vi "Max Nr of Scalar Channels Test.vi"() -> ()   [LabVIEW 2018]
panel:
  in  "I16 4":i16
  in  "I8 4":i8
  in  "I64 4":i64
  in  "I32 4":i32
  out "I16 out 4":i16
  out "I8 out 4":i8
  out "I32 out 4":i32
  in  "Group1.I16 3":i16
  in  "Group1.I8 3":i8
  in  "Group1.I64 3":i64
  in  "Group1.I32 3":i32
  in  "Group1.U16 3":u16
  in  "Group1.U8 3":u8
  in  "Group1.U64 3":u64
  in  "Group1.U32 3":u32
  in  "Group1.SGL 3":sgl
  in  "Group2.Boolean 3":bool
  out "Group1.I16 out 3":i16
  out "Group1.I8 out 3":i8
  out "Group1.I64 out 3":i64
  out "Group1.I32 out 3":i32
  out "Group1.U16 out 3":u16
  out "Group1.U8 out 3":u8
  out "Group1.U64 out 3":u64
  out "Group1.U32 out 3":u32
  out "Group1.SGL out 3":sgl
  out "Group2.Boolean out 3":bool
  in  "Group2.FXP24.5 3":fxp<+/-,24,5>
  in  "Group2.FXP16.5 3":fxp<+/-,16,5>
  in  "Group2.FXP32.8 3":fxp<+/-,32,8>
  in  "Group2.FXP64.32 3":fxp<+/-,64,32>
  out "Group2.FXP24.5 out 3":fxp<+/-,24,5>
  out "Group2.FXP16.5 out 3":fxp<+/-,16,5>
  out "Group2.FXP32.8 out 3":fxp<+/-,32,8>
  out "Group2.FXP64.32 out 3":fxp<+/-,64,32>
  in  "Group2.FXP16.7 3":fxp<+/-,16,7>
  out "Group2.FXP16.7 out 3":fxp<+/-,16,7>
  in  "Group2.FXP20.5 3":fxp<+/-,20,5>
  out "Group2.FXP20.5 out 3":fxp<+/-,20,5>
  in  "Group2.FXP27.5 3":fxp<+/-,27,5>
  out "Group2.FXP27.5 out 3":fxp<+/-,27,5>
  in  "Group2.FXP32.16 3":fxp<+/-,32,16>
  out "Group2.FXP32.16 out 3":fxp<+/-,32,16>
  in  "Group2.FXP16.3 3":fxp<+,16,3>
  out "Group2.FXP16.3 out 3":fxp<+,16,3>
  in  "Group2.FXP18.3 3":fxp<+,18,3>
  out "Group2.FXP18.3 out 3":fxp<+,18,3>
  in  "I16 3":i16
  in  "I8 3":i8
  in  "I64 3":i64
  in  "I32 3":i32
  in  "U16 3":u16
  in  "U8 3":u8
  in  "U64 3":u64
  in  "U32 3":u32
  in  "SGL 3":sgl
  in  "Boolean 3":bool
  out "I16 out 3":i16
  out "I8 out 3":i8
  out "I64 out 3":i64
  out "I32 out 3":i32
  out "U16 out 3":u16
  out "U8 out 3":u8
  out "U64 out 3":u64
  out "U32 out 3":u32
  out "SGL out 3":sgl
  out "Boolean out 3":bool
  in  "FXP24.5 3":fxp<+/-,24,5>
  in  "FXP16.5 3":fxp<+/-,16,5>
  in  "FXP32.8 3":fxp<+/-,32,8>
  in  "FXP64.32 3":fxp<+/-,64,32>
  out "FXP24.5 out 3":fxp<+/-,24,5>
  out "FXP16.5 out 3":fxp<+/-,16,5>
  out "FXP32.8 out 3":fxp<+/-,32,8>
  out "FXP64.32 out 3":fxp<+/-,64,32>
  in  "FXP16.7 3":fxp<+/-,16,7>
  out "FXP16.7 out 3":fxp<+/-,16,7>
  in  "FXP20.5 3":fxp<+/-,20,5>
  out "FXP20.5 out 3":fxp<+/-,20,5>
  in  "FXP27.5 3":fxp<+/-,27,5>
  out "FXP27.5 out 3":fxp<+/-,27,5>
  in  "FXP32.16 3":fxp<+/-,32,16>
  out "FXP32.16 out 3":fxp<+/-,32,16>
  in  "FXP16.3 3":fxp<+,16,3>
  out "FXP16.3 out 3":fxp<+,16,3>
  in  "FXP18.3 3":fxp<+,18,3>
  out "FXP18.3 out 3":fxp<+,18,3>
  in  "Group1.I16 2":i16
  in  "Group1.I8 2":i8
  in  "Group1.I64 2":i64
  in  "Group1.I32 2":i32
  in  "Group1.U16 2":u16
  in  "Group1.U8 2":u8
  in  "Group1.U64 2":u64
  in  "Group1.U32 2":u32
  in  "Group1.SGL 2":sgl
  in  "Group2.Boolean 2":bool
  out "Group1.I16 out 2":i16
  out "Group1.I8 out 2":i8
  out "Group1.I64 out 2":i64
  out "Group1.I32 out 2":i32
  out "Group1.U16 out 2":u16
  out "Group1.U8 out 2":u8
  out "Group1.U64 out 2":u64
  out "Group1.U32 out 2":u32
  out "Group1.SGL out 2":sgl
  out "Group2.Boolean out 2":bool
  in  "Group2.FXP24.5 2":fxp<+/-,24,5>
  in  "Group2.FXP16.5 2":fxp<+/-,16,5>
  in  "Group2.FXP32.8 2":fxp<+/-,32,8>
  in  "Group2.FXP64.32 2":fxp<+/-,64,32>
  out "Group2.FXP24.5 out 2":fxp<+/-,24,5>
  out "Group2.FXP16.5 out 2":fxp<+/-,16,5>
  out "Group2.FXP32.8 out 2":fxp<+/-,32,8>
  out "Group2.FXP64.32 out 2":fxp<+/-,64,32>
  in  "Group2.FXP16.7 2":fxp<+/-,16,7>
  out "Group2.FXP16.7 out 2":fxp<+/-,16,7>
  in  "Group2.FXP20.5 2":fxp<+/-,20,5>
  out "Group2.FXP20.5 out 2":fxp<+/-,20,5>
  in  "Group2.FXP27.5 2":fxp<+/-,27,5>
  out "Group2.FXP27.5 out 2":fxp<+/-,27,5>
  in  "Group2.FXP32.16 2":fxp<+/-,32,16>
  out "Group2.FXP32.16 out 2":fxp<+/-,32,16>
  in  "Group2.FXP16.3 2":fxp<+,16,3>
  out "Group2.FXP16.3 out 2":fxp<+,16,3>
  in  "Group2.FXP18.3 2":fxp<+,18,3>
  out "Group2.FXP18.3 out 2":fxp<+,18,3>
  in  "I16 2":i16
  in  "I8 2":i8
  in  "I64 2":i64
  in  "I32 2":i32
  in  "U16 2":u16
  in  "U8 2":u8
  in  "U64 2":u64
  in  "U32 2":u32
  in  "SGL 2":sgl
  in  "Boolean 2":bool
  out "I16 out 2":i16
  out "I8 out 2":i8
  out "I64 out 2":i64
  out "I32 out 2":i32
  out "U16 out 2":u16
  out "U8 out 2":u8
  out "U64 out 2":u64
  out "U32 out 2":u32
  out "SGL out 2":sgl
  out "Boolean out 2":bool
  in  "FXP24.5 2":fxp<+/-,24,5>
  in  "FXP16.5 2":fxp<+/-,16,5>
  in  "FXP32.8 2":fxp<+/-,32,8>
  in  "FXP64.32 2":fxp<+/-,64,32>
  out "FXP24.5 out 2":fxp<+/-,24,5>
  out "FXP16.5 out 2":fxp<+/-,16,5>
  out "FXP32.8 out 2":fxp<+/-,32,8>
  out "FXP64.32 out 2":fxp<+/-,64,32>
  in  "FXP16.7 2":fxp<+/-,16,7>
  out "FXP16.7 out 2":fxp<+/-,16,7>
  in  "FXP20.5 2":fxp<+/-,20,5>
  out "FXP20.5 out 2":fxp<+/-,20,5>
  in  "FXP27.5 2":fxp<+/-,27,5>
  out "FXP27.5 out 2":fxp<+/-,27,5>
  in  "FXP32.16 2":fxp<+/-,32,16>
  out "FXP32.16 out 2":fxp<+/-,32,16>
  in  "FXP16.3 2":fxp<+,16,3>
  out "FXP16.3 out 2":fxp<+,16,3>
  in  "FXP18.3 2":fxp<+,18,3>
  out "FXP18.3 out 2":fxp<+,18,3>
  in  "Group1.I16":i16
  in  "Group1.I8":i8
  in  "Group1.I64":i64
  in  "Group1.I32":i32
  in  "Group1.U16":u16
  in  "Group1.U8":u8
  in  "Group1.U64":u64
  in  "Group1.U32":u32
  in  "Group1.SGL":sgl
  in  "Group2.Boolean":bool
  out "Group1.I16 out":i16
  out "Group1.I8 out":i8
  out "Group1.I64 out":i64
  out "Group1.I32 out":i32
  out "Group1.U16 out":u16
  out "Group1.U8 out":u8
  out "Group1.U64 out":u64
  out "Group1.U32 out":u32
  out "Group1.SGL out":sgl
  out "Group2.Boolean out":bool
  in  "Group2.FXP24.5":fxp<+/-,24,5>
  in  "Group2.FXP16.5":fxp<+/-,16,5>
  in  "Group2.FXP32.8":fxp<+/-,32,8>
  in  "Group2.FXP64.32":fxp<+/-,64,32>
  out "Group2.FXP24.5 out":fxp<+/-,24,5>
  out "Group2.FXP16.5 out":fxp<+/-,16,5>
  out "Group2.FXP32.8 out":fxp<+/-,32,8>
  out "Group2.FXP64.32 out":fxp<+/-,64,32>
  in  "Group2.FXP16.7":fxp<+/-,16,7>
  out "Group2.FXP16.7 out":fxp<+/-,16,7>
  in  "Group2.FXP20.5":fxp<+/-,20,5>
  out "Group2.FXP20.5 out":fxp<+/-,20,5>
  in  "Group2.FXP27.5":fxp<+/-,27,5>
  out "Group2.FXP27.5 out":fxp<+/-,27,5>
  in  "Group2.FXP32.16":fxp<+/-,32,16>
  out "Group2.FXP32.16 out":fxp<+/-,32,16>
  in  "Group2.FXP16.3":fxp<+,16,3>
  out "Group2.FXP16.3 out":fxp<+,16,3>
  in  "Group2.FXP18.3":fxp<+,18,3>
  out "Group2.FXP18.3 out":fxp<+,18,3>
  in  "FXP18.3":fxp<+,18,3>
  out "FXP18.3 out":fxp<+,18,3>
  in  "FXP16.3":fxp<+,16,3>
  out "FXP16.3 out":fxp<+,16,3>
  in  "FXP32.16":fxp<+/-,32,16>
  out "FXP32.16 out":fxp<+/-,32,16>
  in  "FXP27.5":fxp<+/-,27,5>
  out "FXP27.5 out":fxp<+/-,27,5>
  in  "FXP20.5":fxp<+/-,20,5>
  out "FXP20.5 out":fxp<+/-,20,5>
  in  "FXP16.7":fxp<+/-,16,7>
  out "FXP16.7 out":fxp<+/-,16,7>
  out "FXP64.32 out":fxp<+/-,64,32>
  out "FXP32.8 out":fxp<+/-,32,8>
  out "FXP16.5 out":fxp<+/-,16,5>
  out "FXP24.5 out":fxp<+/-,24,5>
  in  "FXP64.32":fxp<+/-,64,32>
  in  "FXP32.8":fxp<+/-,32,8>
  in  "FXP16.5":fxp<+/-,16,5>
  in  "FXP24.5":fxp<+/-,24,5>
  in  "I16":i16
  in  "I8":i8
  in  "I64":i64
  in  "I32":i32
  in  "U16":u16
  in  "U8":u8
  in  "U64":u64
  in  "U32":u32
  in  "SGL":sgl
  in  "Boolean":bool
  out "I16 out":i16
  out "I8 out":i8
  out "I64 out":i64
  out "I32 out":i32
  out "U16 out":u16
  out "U8 out":u8
  out "U64 out":u64
  out "U32 out":u32
  out "SGL out":sgl
  out "Boolean out":bool
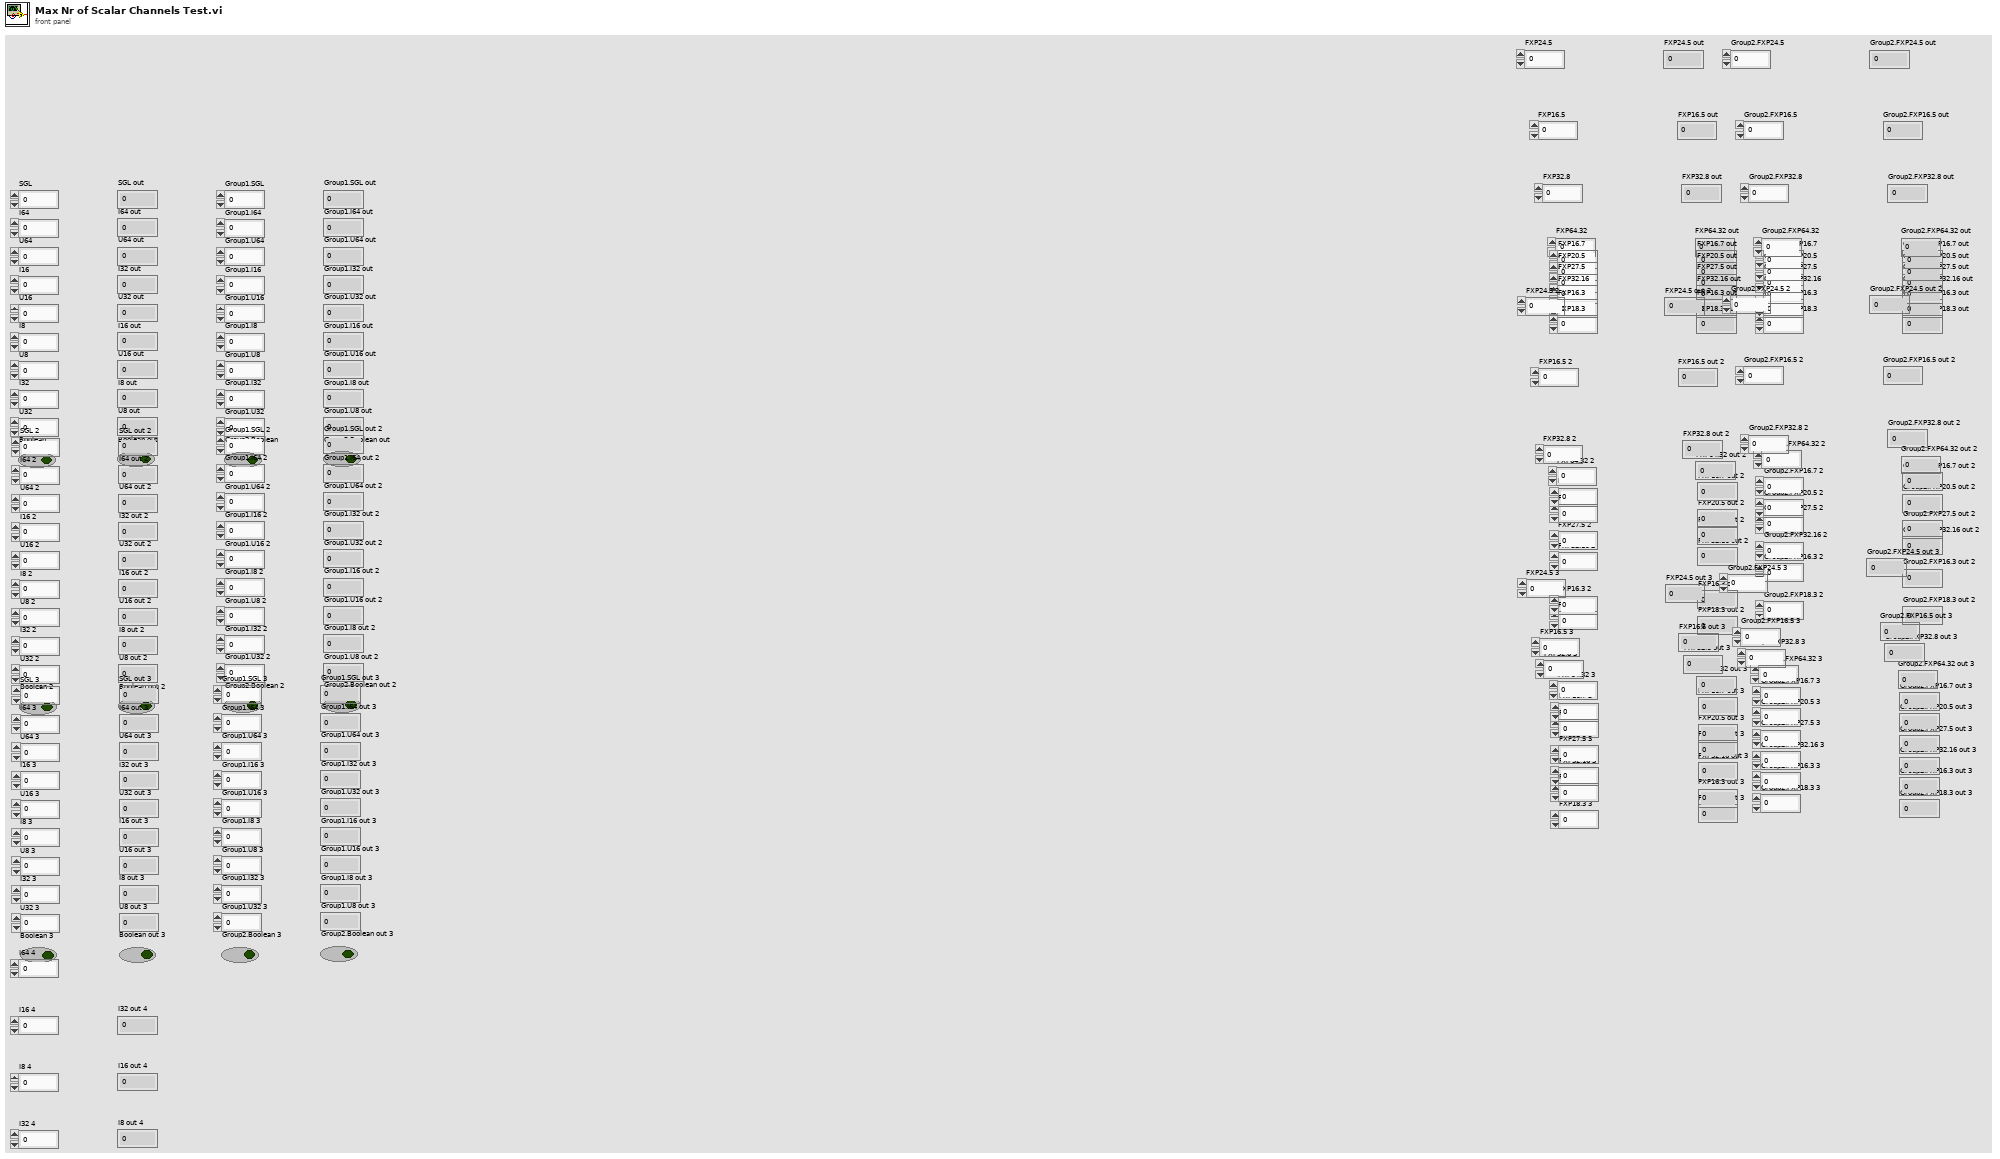
[diagram p1: front panel]
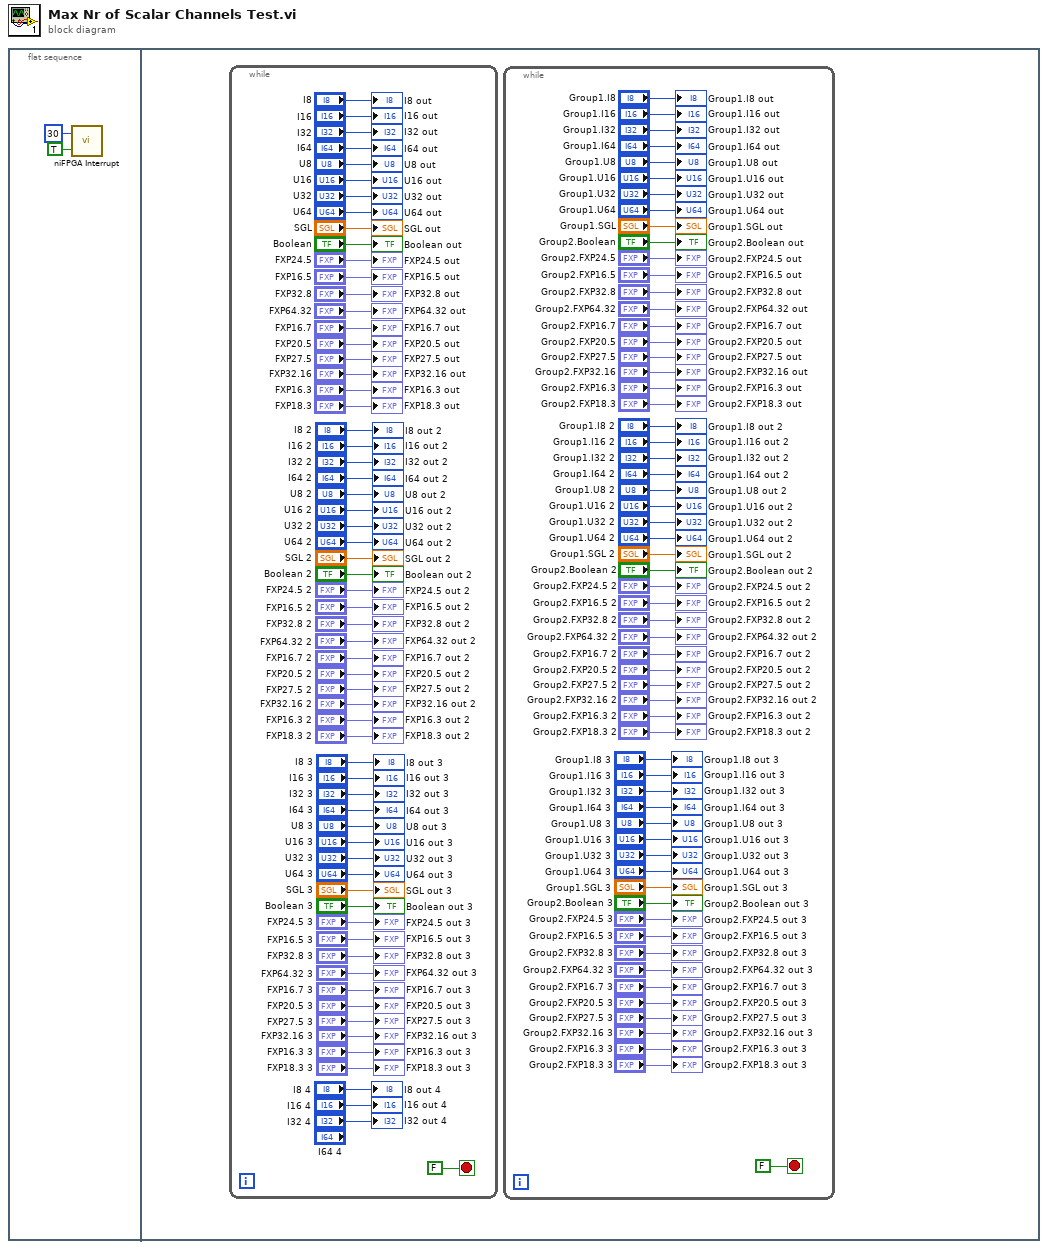
[diagram p0: block diagram]
diagram:
  n1 = flat-sequence {
    frame #0 {
      n2 = call <vilib>:"niFPGA Interrupt.vi"("Wait Until Cleared (F)"=TRUE, "IRQ Number (0)"=u8 30) -> ()  [unwired: 1 in]
    }
    frame #1 {
      n3 = while {
        stop <- FALSE stop-if-true
        "I16 out" <- "I16"
        "I8 out" <- "I8"
        "I64 out" <- "I64"
        "I32 out" <- "I32"
        "U16 out" <- "U16"
        "U8 out" <- "U8"
        "U64 out" <- "U64"
        "U32 out" <- "U32"
        "SGL out" <- "SGL"
        "Boolean out" <- "Boolean"
        "FXP24.5 out" <- "FXP24.5"
        "FXP16.5 out" <- "FXP16.5"
        "FXP32.8 out" <- "FXP32.8"
        "FXP64.32 out" <- "FXP64.32"
        "FXP16.7 out" <- "FXP16.7"
        "FXP20.5 out" <- "FXP20.5"
        "FXP27.5 out" <- "FXP27.5"
        "FXP32.16 out" <- "FXP32.16"
        "FXP16.3 out" <- "FXP16.3"
        "FXP18.3 out" <- "FXP18.3"
        "I16 out 2" <- "I16 2"
        "I8 out 2" <- "I8 2"
        "I64 out 2" <- "I64 2"
        "I32 out 2" <- "I32 2"
        "U16 out 2" <- "U16 2"
        "U8 out 2" <- "U8 2"
        "U64 out 2" <- "U64 2"
        "U32 out 2" <- "U32 2"
        "SGL out 2" <- "SGL 2"
        "Boolean out 2" <- "Boolean 2"
        "FXP24.5 out 2" <- "FXP24.5 2"
        "FXP16.5 out 2" <- "FXP16.5 2"
        "FXP32.8 out 2" <- "FXP32.8 2"
        "FXP64.32 out 2" <- "FXP64.32 2"
        "FXP16.7 out 2" <- "FXP16.7 2"
        "FXP20.5 out 2" <- "FXP20.5 2"
        "FXP27.5 out 2" <- "FXP27.5 2"
        "FXP32.16 out 2" <- "FXP32.16 2"
        "FXP16.3 out 2" <- "FXP16.3 2"
        "FXP18.3 out 2" <- "FXP18.3 2"
        "I16 out 3" <- "I16 3"
        "I8 out 3" <- "I8 3"
        "I64 out 3" <- "I64 3"
        "I32 out 3" <- "I32 3"
        "U16 out 3" <- "U16 3"
        "U8 out 3" <- "U8 3"
        "U64 out 3" <- "U64 3"
        "U32 out 3" <- "U32 3"
        "SGL out 3" <- "SGL 3"
        "Boolean out 3" <- "Boolean 3"
        "FXP24.5 out 3" <- "FXP24.5 3"
        "FXP16.5 out 3" <- "FXP16.5 3"
        "FXP32.8 out 3" <- "FXP32.8 3"
        "FXP64.32 out 3" <- "FXP64.32 3"
        "FXP16.7 out 3" <- "FXP16.7 3"
        "FXP20.5 out 3" <- "FXP20.5 3"
        "FXP27.5 out 3" <- "FXP27.5 3"
        "FXP32.16 out 3" <- "FXP32.16 3"
        "FXP16.3 out 3" <- "FXP16.3 3"
        "FXP18.3 out 3" <- "FXP18.3 3"
        "I16 out 4" <- "I16 4"
        "I8 out 4" <- "I8 4"
        "I32 out 4" <- "I32 4"
      }
      n4 = while {
        stop <- FALSE stop-if-true
        "Group1.I16 out" <- "Group1.I16"
        "Group1.I8 out" <- "Group1.I8"
        "Group1.I64 out" <- "Group1.I64"
        "Group1.I32 out" <- "Group1.I32"
        "Group1.U16 out" <- "Group1.U16"
        "Group1.U8 out" <- "Group1.U8"
        "Group1.U64 out" <- "Group1.U64"
        "Group1.U32 out" <- "Group1.U32"
        "Group1.SGL out" <- "Group1.SGL"
        "Group2.Boolean out" <- "Group2.Boolean"
        "Group2.FXP24.5 out" <- "Group2.FXP24.5"
        "Group2.FXP16.5 out" <- "Group2.FXP16.5"
        "Group2.FXP32.8 out" <- "Group2.FXP32.8"
        "Group2.FXP64.32 out" <- "Group2.FXP64.32"
        "Group2.FXP16.7 out" <- "Group2.FXP16.7"
        "Group2.FXP20.5 out" <- "Group2.FXP20.5"
        "Group2.FXP27.5 out" <- "Group2.FXP27.5"
        "Group2.FXP32.16 out" <- "Group2.FXP32.16"
        "Group2.FXP16.3 out" <- "Group2.FXP16.3"
        "Group2.FXP18.3 out" <- "Group2.FXP18.3"
        "Group1.I16 out 2" <- "Group1.I16 2"
        "Group1.I8 out 2" <- "Group1.I8 2"
        "Group1.I64 out 2" <- "Group1.I64 2"
        "Group1.I32 out 2" <- "Group1.I32 2"
        "Group1.U16 out 2" <- "Group1.U16 2"
        "Group1.U8 out 2" <- "Group1.U8 2"
        "Group1.U64 out 2" <- "Group1.U64 2"
        "Group1.U32 out 2" <- "Group1.U32 2"
        "Group1.SGL out 2" <- "Group1.SGL 2"
        "Group2.Boolean out 2" <- "Group2.Boolean 2"
        "Group2.FXP24.5 out 2" <- "Group2.FXP24.5 2"
        "Group2.FXP16.5 out 2" <- "Group2.FXP16.5 2"
        "Group2.FXP32.8 out 2" <- "Group2.FXP32.8 2"
        "Group2.FXP64.32 out 2" <- "Group2.FXP64.32 2"
        "Group2.FXP16.7 out 2" <- "Group2.FXP16.7 2"
        "Group2.FXP20.5 out 2" <- "Group2.FXP20.5 2"
        "Group2.FXP27.5 out 2" <- "Group2.FXP27.5 2"
        "Group2.FXP32.16 out 2" <- "Group2.FXP32.16 2"
        "Group2.FXP16.3 out 2" <- "Group2.FXP16.3 2"
        "Group2.FXP18.3 out 2" <- "Group2.FXP18.3 2"
        "Group1.I16 out 3" <- "Group1.I16 3"
        "Group1.I8 out 3" <- "Group1.I8 3"
        "Group1.I64 out 3" <- "Group1.I64 3"
        "Group1.I32 out 3" <- "Group1.I32 3"
        "Group1.U16 out 3" <- "Group1.U16 3"
        "Group1.U8 out 3" <- "Group1.U8 3"
        "Group1.U64 out 3" <- "Group1.U64 3"
        "Group1.U32 out 3" <- "Group1.U32 3"
        "Group1.SGL out 3" <- "Group1.SGL 3"
        "Group2.Boolean out 3" <- "Group2.Boolean 3"
        "Group2.FXP24.5 out 3" <- "Group2.FXP24.5 3"
        "Group2.FXP16.5 out 3" <- "Group2.FXP16.5 3"
        "Group2.FXP32.8 out 3" <- "Group2.FXP32.8 3"
        "Group2.FXP64.32 out 3" <- "Group2.FXP64.32 3"
        "Group2.FXP16.7 out 3" <- "Group2.FXP16.7 3"
        "Group2.FXP20.5 out 3" <- "Group2.FXP20.5 3"
        "Group2.FXP27.5 out 3" <- "Group2.FXP27.5 3"
        "Group2.FXP32.16 out 3" <- "Group2.FXP32.16 3"
        "Group2.FXP16.3 out 3" <- "Group2.FXP16.3 3"
        "Group2.FXP18.3 out 3" <- "Group2.FXP18.3 3"
      }
    }
  }
